vi "Measure.vi"(0 "VISA resource name":refnum<visa-resource-name>, 1 "Baud rate (115200)":u32=115200 min=38400 max=500000 step=1, 3 "Initial Tare":sgl[](array[numeric]), 4 "Motor relative position":dbl(knob) min=0.0 max=199.9 scale=0.0..199.9, 5 "Samples per position":i32, 6 "Direction":bool, 8 "error in":errorcluster, 11 "Cal Param":sgl[](array[numeric])) -> (12 "Motor Ready":bool, 14 "Monitor":T2, 15 "Measure":T1, 16 "error out":errorcluster, 17 "VISA resource name out":refnum<visa-resource-name>, 18 "Communication\nAcknowledged":bool, 19 "Progress":u8(slide) scale=0.0..100.0)   [LabVIEW 2018]
uses:
  Progress.vi
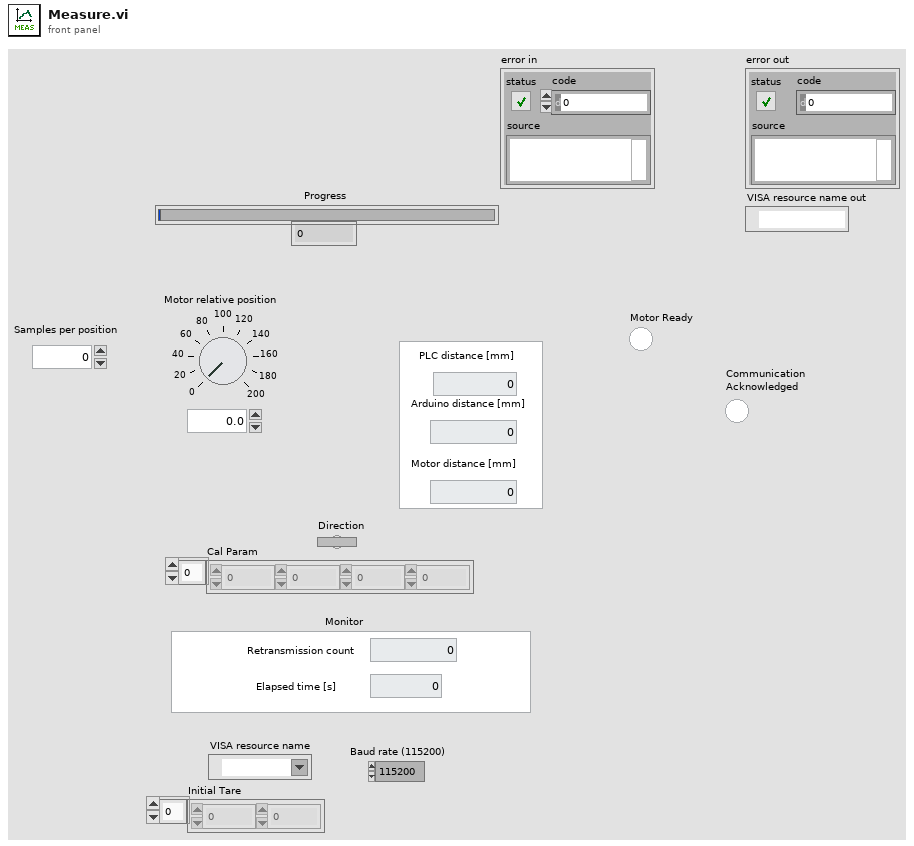
[diagram p1: front panel]
types:
  T1 = cluster{"PLC distance [mm] ":dbl, "Arduino distance [mm]":dbl, "Motor distance [mm]":dbl}
  T2 = cluster{"Elapsed time [s]":dbl, "Retransmission count":dbl}
  T3 = cluster{"PLC Sensor":dbl, "Arduino Sensor":dbl, "Position Reference":dbl}
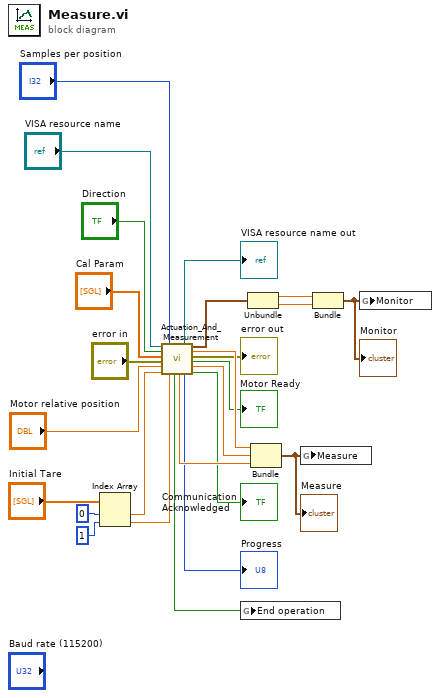
[diagram p0: block diagram]
diagram:
  n1 = Index Array(array="Initial Tare", index #1=0 ("index"), index #2=1 ("index")) -> (element #1=w9:sgl, element #2=w8:sgl)
  n2 = call "Actuation_And_Measurement.vi"("VISA resource name"="VISA resource name", "Direction"="Direction", "Cal Param"="Cal Param", "error in (no error)"="error in", "Motor relative position"="Motor relative position", "Zero Offset"=w9, "Samples per position"="Samples per position", "Fullscale"=w8) -> ("End operation"=w3:bool, "Position Reference"=w24:dbl, "VISA resource name out"=→"VISA resource name out":refnum<visa-resource-name>, "Progress"=→"Progress":u8, "Monitor"=w23:T2, "PLC Sensor"=w20:dbl, "error out"=→"error out":errorcluster, "Motor Ready"=→"Motor Ready":bool, "Arduino Sensor"=w19:dbl, "Communication\nAcknowledged"=→"Communication\nAcknowledged":bool)  [unwired: 2 in]
  n3 = global write "Progress.vi" "End operation"(w3) -> ()
  n4 = Unbundle(w23) -> ("Elapsed time [s]"=w22:dbl, "Retransmission count"=w21:dbl)
  n5 = Bundle("PLC Sensor"=w20, "Arduino Sensor"=w19, "Position Reference"=w24) -> (w2:T3)  [unwired: 1 in]
  "Measure" <- w2
  n6 = global write "Progress.vi" "Measure"(w2) -> ()
  n7 = Bundle("Elapsed time [s]"=w22, "Retransmission count"=w21) -> (w1:T2)  [unwired: 1 in]
  "Monitor" <- w1
  n8 = global write "Progress.vi" "Monitor"(w1) -> ()
